vi "Example.vi"() -> ()   [LabVIEW 2016]
uses:
  Data Def/ASDA-A2_Connection Data.ctl
panel:
  out "DI Status":T1
  out "Position":cluster{"CN2 Encoder":i32, "CN5 Encoder":i32}
  out "Sevro Status":T2
  in  "Monitor":bool
  in  "Server On/Off":bool
  out "State":bool
  in  "Setting Tab":enum32{"Motor Home Setting", "Jog", "PR Mode"}(tab)
  in  "Motor Home Setting":T3={"Reach Limit"=enum."Return", "Z Phase"=enum."Ignore", "Direction"=enum."Negative+DI Limit", "First High Speed(0.1RPM)"=1000, "Second Low Speed(0.1RPM)"=200, "Home Position"=0}
  in  "Jog":bool
  in  "Jog(RPM)":u32
  in  "Jog Type":enum16{"CCW", "CW"}(ring)
  in  "PR Start":bool
  in  "PR Motor Home":bool
  in  "PR Stop":bool
  in  "Path Setting":T4={"Command"=enum."Absolute", "Position"=1000, "Speed"=1000}
  in  "Connect":bool
  in  "Connection Data":T5={"COM Port"="COM6", "Baud Rate"=19200, "Unit ID"=1}
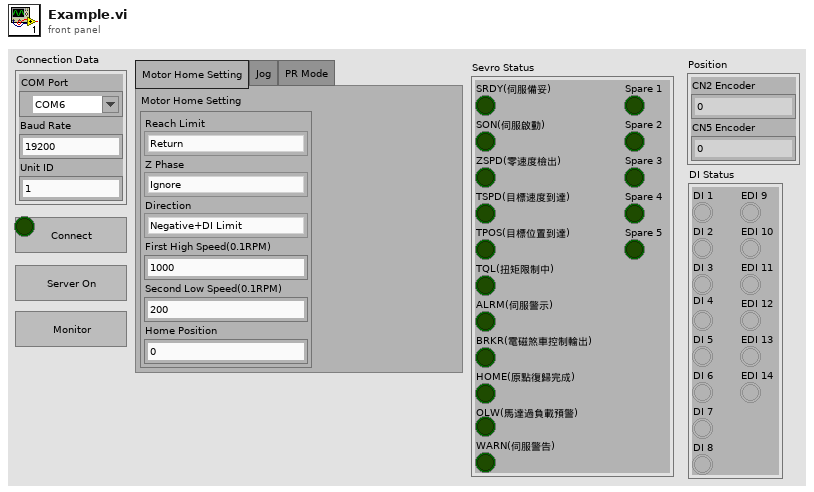
[diagram p1: front panel]
types:
  T1 = cluster{"DI 1":bool, "DI 2":bool, "DI 3":bool, "DI 4":bool, "DI 5":bool, "DI 6":bool, "DI 7":bool, "DI 8":bool, "EDI 9":bool, "EDI 10":bool, "EDI 11":bool, "EDI 12":bool, "EDI 13":bool, "EDI 14":bool}
  T2 = cluster{"SRDY(伺服備妥)":bool, "SON(伺服啟動)":bool, "ZSPD(零速度檢出)":bool, "TSPD(目標速度到達)":bool, "TPOS(目標位置到達)":bool, "TQL(扭矩限制中)":bool, "ALRM(伺服警示)":bool, "BRKR(電磁煞車控制輸出)":bool, "HOME(原點復歸完成)":bool, "OLW(馬達過負載預警)":bool, "WARN(伺服警告)":bool, "Spare 1":bool, "Spare 2":bool, "Spare 3":bool, "Spare 4":bool, "Spare 5":bool}
  T3 = cluster{"Reach Limit":enum8{"Alarm", "Return"}, "Z Phase":enum8{"Return", "Forward", "Ignore"}, "Direction":enum8{"Position", "Negative", "Position+DI OFF->ON  Limit", "Negative+DI OFF->ON Limit", "Position+Find Z", "Negative+Find Z", "Position+DI ON->OFF  Limit", "Negative+DI ON->OFF  Limit", "Location ORG", "Position+DI Limit", "Negative+DI Limit"}, "First High Speed(0.1RPM)":u32, "Second Low Speed(0.1RPM)":u32, "Home Position":i32}
  T4 = cluster{"Command":enum16{"Absolute", "Increase", "Relative"}, "Position":i32, "Speed":u16}
  T5 = typedef "ASDA-A2_Connection Data.ctl" = cluster{"COM Port":refnum<visa-resource-name>, "Baud Rate":u32, "Unit ID":u8}
  T6 = typedef "ASDA-A2_Buffer Data.ctl" = cluster{"DVR Refnum":refnum<data-value>}
  T7 = cluster{"SRDY":bool, "SON":bool, "ZSPD":bool, "TSPD":bool, "TPOS":bool, "TQL":bool, "ALRM":bool, "BRKR":bool, "HOME":bool, "OLW":bool, "WARN":bool, "Spare 1":bool, "Spare 2":bool, "Spare 3":bool, "Spare 4":bool, "Spare 5":bool}
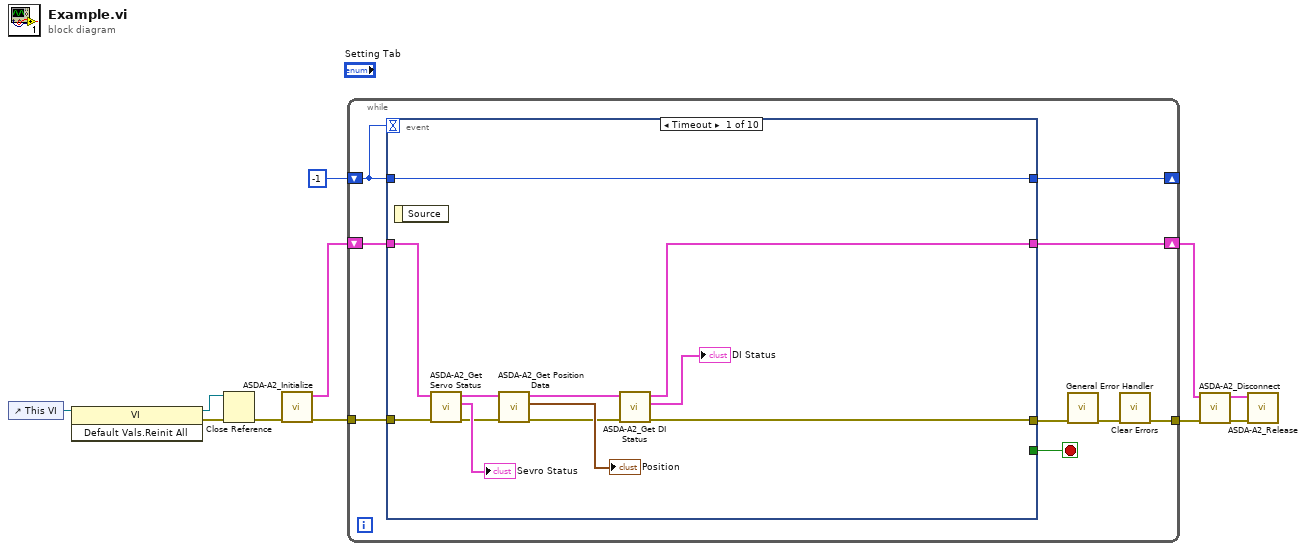
[diagram p0: block diagram]
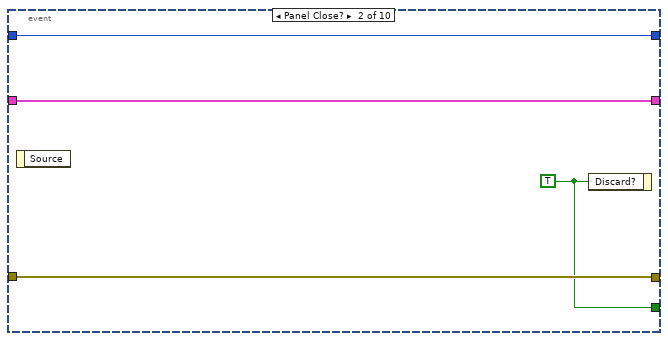
[diagram p2: hidden frame]
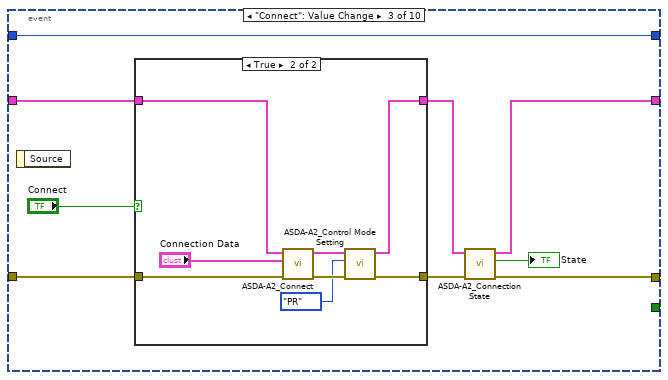
[diagram p3: hidden frame]
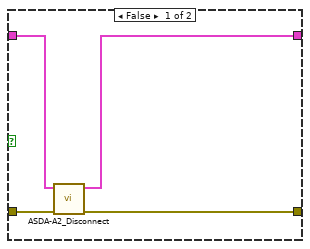
[diagram p4: hidden frame]
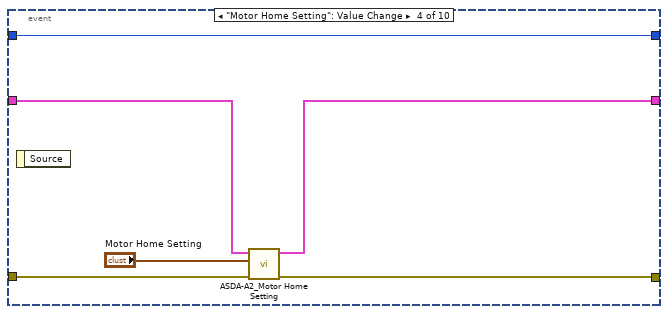
[diagram p5: hidden frame]
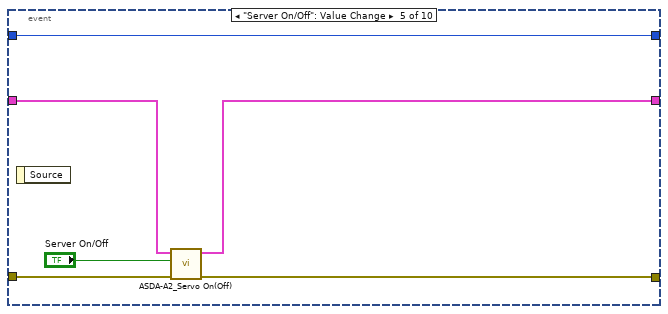
[diagram p6: hidden frame]
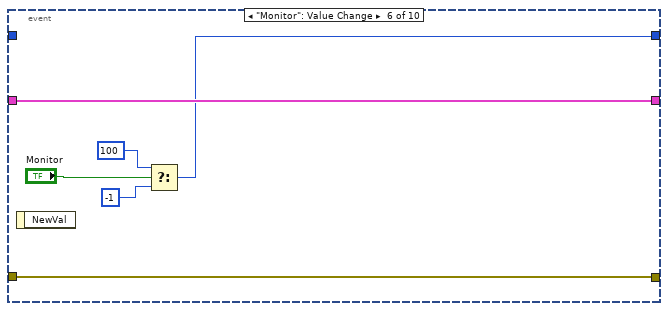
[diagram p7: hidden frame]
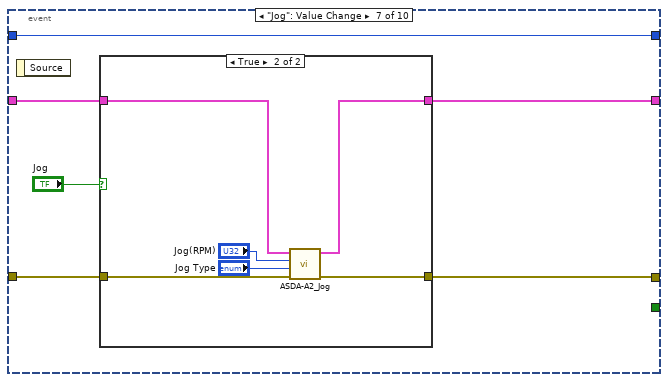
[diagram p8: hidden frame]
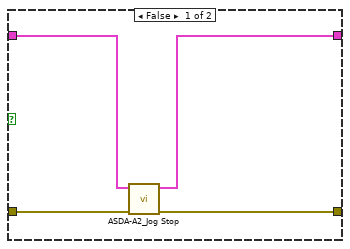
[diagram p9: hidden frame]
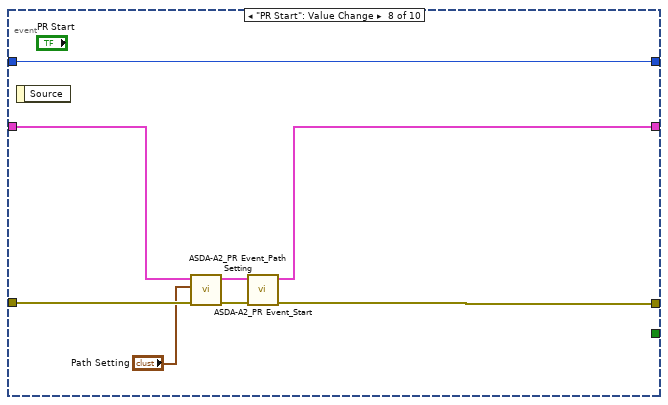
[diagram p10: hidden frame]
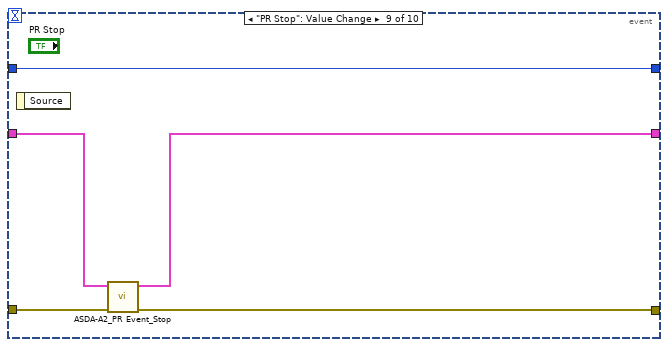
[diagram p11: hidden frame]
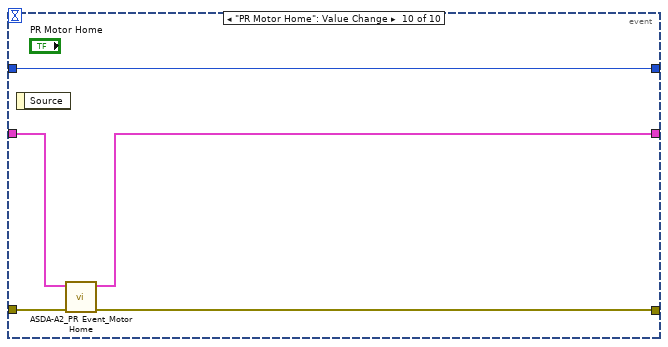
[diagram p12: hidden frame]
diagram:
  n1 = control-ref of="This VI"() -> (w6:refnum<vi>)
  n2 = invoke class="VI" method="Default Vals.Reinit All"(reference=w6) -> (reference out=w3:refnum<vi>, error out=w4:errorcluster)  [unwired: 2 in, 1 out]
  n3 = Close Reference(reference=w3, error in (no error)=w4) -> (error out=w5:errorcluster)
  n4 = call "ASDA-A2_Initialize.vi"("error in"=w5) -> ("error out"=w11:errorcluster, "Buffer Data"=w10:T6)  [unwired: 9 in]
  n5 = while {
    tunnel: w11 -> [w20]
    tunnel: [w14] -> w9
    shift-right: [w16] -> w8
    shift-left: w10 -> [w19]
    shift-right: [w12] -> _
    shift-left: -1 -> [w13]
    stop <- w18 stop-if-true
    n6 = event shown="[0] Timeout" {
      selector: _ -> [_ _ _ _ _ _ _ _ _ _]
      dyn-events: _ -> [_ _ _ _ _ _ _ _ _ _]
      timeout: w13 -> [_ _ _ _ _ _ _ _ _ _]
      tunnel: w20 -> [w30 w36 w45 w62 w69 w73 w78 w97 w103 w108]
      tunnel: w19 -> [w31 w34 w44 w61 w68 w75 w80 w94 w102 w107]
      tunnel: [w23 w36 w40 w59 w66 w73 w77 w98 w100 w105] -> w17
      tunnel: [_ w35 _ _ _ _ _ _ _ _] -> w18
      tunnel: [w22 w34 w41 w60 w67 w75 w76 w93 w101 w106] -> w16
      tunnel: w13 -> [w32 w33 w37 w58 w64 _ w81 w99 w104 w109]
      tunnel: [w32 w33 w37 w58 w64 w70 w81 w99 w104 w109] -> w12
      event Timeout {
        n7 = event-data() -> ()  [unwired: 1 in, 1 out]
        n8 = call "ASDA-A2_Get Servo Status.vi"("error in"=w30, "Buffer Data In"=w31) -> ("error out"=w28:errorcluster, "Sevro Status"=→"Sevro Status":T7, "Buffer Data Out"=w27:T6)  [unwired: 7 in]
        n9 = call "ASDA-A2_Get Position Data.vi"("error in"=w28, "Buffer Data In"=w27) -> ("error out"=w25:errorcluster, "Position"=→"Position":cluster{"CN2 Encoder":i32, "CN5 Encoder":i32}, "Buffer Data Out"=w24:T6)  [unwired: 7 in]
        n10 = call "ASDA-A2_Get DI Status.vi"("error in"=w25, "Buffer Data In"=w24) -> ("error out"=w23:errorcluster, "DI Status"=→"DI Status":T1, "Buffer Data Out"=w22:T6)  [unwired: 7 in]
      }
      event Panel Close? {
        w35 = TRUE ("Discard?")
        n11 = event-data() -> ()  [unwired: 1 in, 1 out]
        n12 = event-data("Discard?"=w35) -> ()  [unwired: 1 in, 1 out]
      }
      event "Connect": Value Change {
        n13 = event-data() -> ()  [unwired: 1 in, 1 out]
        n14 = case shown="True" "Connect" {
          tunnel: w45 -> [w49 w56]
          tunnel: w44 -> [w48 w55]
          tunnel: [w47 w51] -> w43
          tunnel: [w46 w50] -> w42
          frame False {
            n15 = call "ASDA-A2_Disconnect.vi"("error in"=w49, "Buffer Data In"=w48) -> ("error out"=w47:errorcluster, "Buffer Data Out"=w46:T6)  [unwired: 8 in]
          }
          frame True {
            n16 = call "ASDA-A2_Connect.vi"("error in"=w56, "Connection Data"="Connection Data", "Buffer Data In"=w55) -> ("error out"=w54:errorcluster, "Buffer Data Out"=w53:T6)  [unwired: 7 in]
            n17 = call "ASDA-A2_Control Mode Setting.vi"("error in"=w54, "Control Mode"=enum32{"PT", "PR", "S", "T", "Sz", "Tz"}."PR", "Buffer Data In"=w53) -> ("error out"=w51:errorcluster, "Buffer Data Out"=w50:T6)  [unwired: 7 in]
          }
        }
        n18 = call "ASDA-A2_Connection State.vi"("error in"=w43, "Buffer Data In"=w42) -> ("error out"=w40:errorcluster, "State Out"=→"State":bool, "Buffer Data Out"=w41:T6)  [unwired: 7 in]
      }
      event "Motor Home Setting": Value Change {
        n19 = event-data() -> ()  [unwired: 1 in, 1 out]
        n20 = call "ASDA-A2_Motor Home Setting.vi"("error in"=w62, "Motor Home Setting"="Motor Home Setting", "Buffer Data In"=w61) -> ("error out"=w59:errorcluster, "Buffer Data Out"=w60:T6)  [unwired: 7 in]
      }
      event "Server On/Off": Value Change {
        n21 = event-data() -> ()  [unwired: 1 in, 1 out]
        n22 = call "ASDA-A2_Servo On(Off).vi"("error in"=w69, "On/Off"="Server On/Off", "Buffer Data In"=w68) -> ("error out"=w66:errorcluster, "Buffer Data Out"=w67:T6)  [unwired: 7 in]
      }
      event "Monitor": Value Change {
        n23 = event-data() -> ()  [unwired: 1 in, 1 out]
        n24 = Select(t=100, s="Monitor", f=-1) -> (s? t:f=w70:i32)
      }
      event "Jog": Value Change {
        n25 = event-data() -> ()  [unwired: 1 in, 1 out]
        n26 = case shown="True" "Jog" {
          tunnel: w80 -> [w83 w87]
          tunnel: w78 -> [w85 w91]
          tunnel: [w84 w90] -> w77
          tunnel: [w82 w86] -> w76
          frame False {
            n27 = call "ASDA-A2_Jog Stop.vi"("error in"=w85, "Buffer Data In"=w83) -> ("error out"=w84:errorcluster, "Buffer Data Out"=w82:T6)  [unwired: 8 in]
          }
          frame True {
            n28 = call "ASDA-A2_Jog.vi"("error in"=w91, "Jog Type"="Jog Type", "Jog(RPM)"="Jog(RPM)", "Buffer Data In"=w87) -> ("error out"=w90:errorcluster, "Buffer Data Out"=w86:T6)  [unwired: 6 in]
          }
        }
      }
      event "PR Start": Value Change {
        n29 = event-data() -> ()  [unwired: 1 in, 1 out]
        n30 = call "ASDA-A2_PR Event_Path Setting.vi"("error in"=w97, "Path Setting"="Path Setting", "Buffer Data In"=w94) -> ("error out"=w96:errorcluster, "Buffer Data Out"=w95:T6)  [unwired: 7 in]
        n31 = call "ASDA-A2_PR Event_Start.vi"("error in"=w96, "Buffer Data In"=w95) -> ("error out"=w98:errorcluster, "Buffer Data Out"=w93:T6)  [unwired: 8 in]
      }
      event "PR Stop": Value Change {
        n32 = event-data() -> ()  [unwired: 1 in, 1 out]
        n33 = call "ASDA-A2_PR Event_Stop.vi"("error in"=w103, "Buffer Data In"=w102) -> ("error out"=w100:errorcluster, "Buffer Data Out"=w101:T6)  [unwired: 8 in]
      }
      event "PR Motor Home": Value Change {
        n34 = event-data() -> ()  [unwired: 1 in, 1 out]
        n35 = call "ASDA-A2_PR Event_Motor Home.vi"("error in"=w108, "Buffer Data In"=w107) -> ("error out"=w105:errorcluster, "Buffer Data Out"=w106:T6)  [unwired: 8 in]
      }
    }
    n36 = call <vilib>:"General Error Handler.vi"("error in (no error)"=w17) -> ("error out"=w15:errorcluster)  [unwired: 10 in, 4 out]
    n37 = call <vilib>:"Clear Errors.vi"("error in (no error)"=w15) -> ("error out"=w14:errorcluster)  [unwired: 5 in, 1 out]
  }
  n38 = call "ASDA-A2_Disconnect.vi"("error in"=w9, "Buffer Data In"=w8) -> ("error out"=w1:errorcluster, "Buffer Data Out"=w2:T6)  [unwired: 8 in]
  n39 = call "ASDA-A2_Release.vi"("error in"=w1, "Buffer Data"=w2) -> ()  [unwired: 9 in, 1 out]
